vi "solar_excel Worksheet Read (Range).vi"(6 "Truncate Empty Cells? (F)":bool, 8 "error in (no error)":errorcluster, 9 "End (1,1 = 'A1')":cluster{"Row":u32, "Column":u32}, 10 "Start (1,1 = 'A1')":cluster{"Row":u32, "Column":u32}, 11 "Excel Worksheet in":T1) -> (0 "error out":errorcluster, 2 "Cells":string[][](array[string]), 3 "Excel Worksheet out":T1)   [LabVIEW 2018]
doc: "This returns a range of cells from the Worksheet specified by the <b>Start</b> and <b>End</b> cell range."
uses:
  solar_excel_ctl Worksheet.ctl
  solar_excel_ctl TSV.ctl
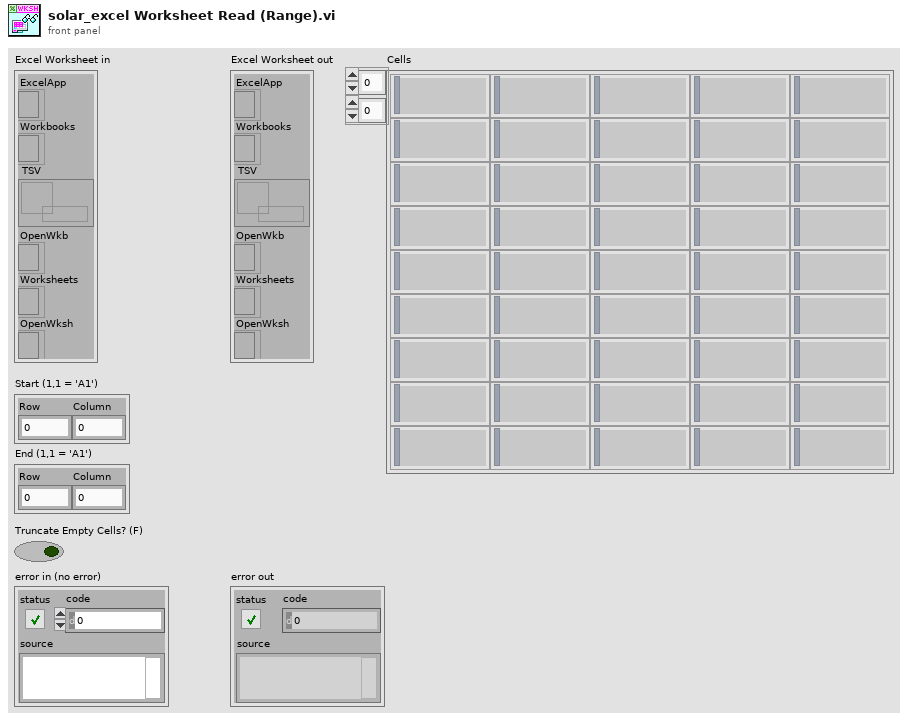
[diagram p1: front panel]
types:
  T1 = typedef "solar_excel_ctl Worksheet.ctl" = cluster{"ExcelApp":refnum<k7>, "Workbooks":refnum<k7>, "TSV":refnum<queue>, "OpenWkb":refnum<k7>, "Worksheets":refnum<k7>, "OpenWksh":refnum<k7>}
  T2 = typedef "solar_excel_ctl TSV.ctl" = cluster{"Path":path, "Dirty":bool, "ActiveSheet":u8, "Worksheets":string[], "Worksheet Cells":cluster{"Cells":string[][]}[]}
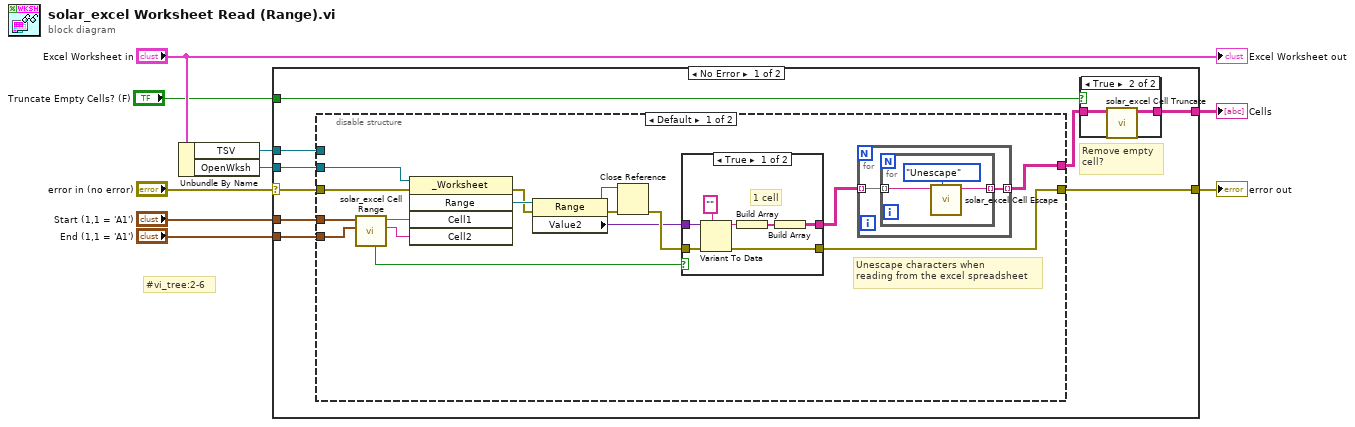
[diagram p0: block diagram]
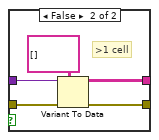
[diagram p2: hidden frame]
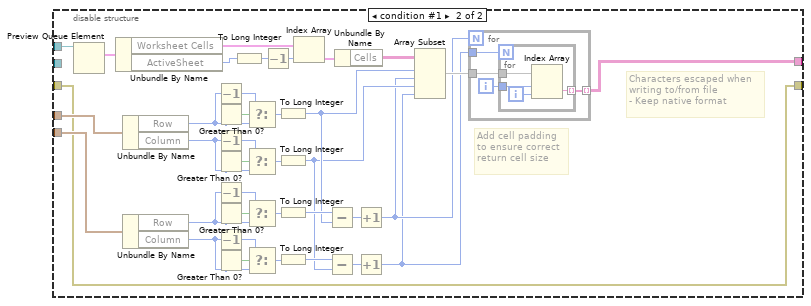
[diagram p3: hidden frame]
diagram:
  # "#vi_tree:2-6"
  n1 = Unbundle By Name("Excel Worksheet in") -> ("TSV"=w1:refnum<queue>, "OpenWksh"=w7:refnum<k7>)
  n2 = case shown="No Error" "error in (no error)" {
    selector: "error in (no error)" -> [w18 w100]
    tunnel: [w16 w100] -> w9
    tunnel: w7 -> [w17 _]
    tunnel: [w13 _] -> w5
    tunnel: "Start (1,1 = 'A1')" -> [w15 _]
    tunnel: "End (1,1 = 'A1')" -> [w14 _]
    tunnel: "Truncate Empty Cells? (F)" -> [w12 _]
    tunnel: w1 -> [w11 _]
    frame No Error {
      # "Remove empty\ncell?"
      n3 = disable-structure shown="Default" {
        disable-tunnel: w18 -> [w33 w56]
        disable-tunnel: w17 -> [w32 _]
        disable-tunnel: [w26 w56] -> w16
        disable-tunnel: w15 -> [w25 w83]
        disable-tunnel: w14 -> [w24 w65]
        disable-tunnel: [w19 w58] -> w10
        disable-tunnel: w11 -> [_ w88]
        frame condition #0 (active) {
          # "Unescape characters when\nreading from the excel spreadsheet"
          n4 = call "solar_excel Cell Range.vi"("End (1,1 = 'A1')"=w24, "Start (1,1 = 'A1')"=w25) -> ("End Cell"=w22:string, "Start Cell"=w23:string, "Same"=w21:bool)  [unwired: 7 in]
          n5 = invoke class="_Worksheet" method="Range"(reference=w32, error in=w33, "Cell1"=w23, "Cell2"=w22) -> (error out=w30:errorcluster, "Range"=w31:refnum<k7>)  [unwired: 1 in, 3 out]
          n6 = property class="Range"(reference=w31, error in=w30) -> (reference out=w28:refnum<k7>, error out=w29:errorcluster, "Value2"=w27:variant)
          n7 = Close Reference(reference=w28, error in (no error)=w29) -> (error out=w34:errorcluster)
          n8 = case shown="True" w21 {
            tunnel: w34 -> [w43 w51]
            tunnel: w27 -> [w44 w50]
            tunnel: [w42 w47] -> w26
            tunnel: [w45 w48] -> w20
            frame True {
              # "1 cell"
              n9 = Variant To Data(error in=w43, type="", Variant=w44) -> (data=w40:string, error out=w42:errorcluster)
              n10 = Build Array(w40) -> (w46:string[])
              n11 = Build Array(w46) -> (w45:string[][])
            }
            frame False {
              # ">1 cell"
              n12 = Variant To Data(error in=w51, type=string[][] [], Variant=w50) -> (data=w48:string[][], error out=w47:errorcluster)
            }
          }
          n13 = for {
            tunnel: w20 -> [w36] mode=indexing
            tunnel: [w35] -> w19 mode=indexing
            n14 = for {
              tunnel: w36 -> [w39] mode=indexing
              tunnel: [w37] -> w35 mode=indexing
              n15 = call "solar_excel Cell Escape.vi"("Action (Escape)"=enum8{"Escape", "Unescape"}."Unescape", "String in"=w39) -> ("String out"=w37:string)  [unwired: 9 in]
            }
          }
        }
        frame condition #1 {
          # "Characters escaped when\nwriting to/from file\n- Keep native format"
          # "Add cell padding\nto ensure correct\nreturn cell size"
          n16 = Preview Queue Element(queue=w88) -> (element=w87:T2)  [unwired: 2 in, 3 out]
          n17 = Unbundle By Name(w87) -> ("Worksheet Cells"=w86:cluster{"Cells":string[][]}[], "ActiveSheet"=w85:u8)
          n18 = Unbundle By Name(w83) -> ("Row"=w79:u32, "Column"=w76:u32)
          n19 = Unbundle By Name(w65) -> ("Row"=w68:u32, "Column"=w71:u32)
          n20 = Decrement(x=w79) -> (x-1=w80:u32)
          n21 = Greater Than 0?(x=w79) -> (x > 0?=w81:bool)
          n22 = Decrement(x=w76) -> (x-1=w78:u32)
          n23 = Greater Than 0?(x=w76) -> (x > 0?=w77:bool)
          n24 = Decrement(x=w68) -> (x-1=w67:u32)
          n25 = Greater Than 0?(x=w68) -> (x > 0?=w66:bool)
          n26 = Decrement(x=w71) -> (x-1=w69:u32)
          n27 = Greater Than 0?(x=w71) -> (x > 0?=w70:bool)
          n28 = To Long Integer(number=w85) -> (32bit integer=w55:i32)
          n29 = Select(t=w80, s=w81, f=w79) -> (s? t:f=w75:u32)
          n30 = Select(t=w78, s=w77, f=w76) -> (s? t:f=w74:u32)
          n31 = Select(t=w67, s=w66, f=w68) -> (s? t:f=w72:u32)
          n32 = Select(t=w69, s=w70, f=w71) -> (s? t:f=w73:u32)
          n33 = Decrement(x=w55) -> (x-1=w54:i32)
          n34 = To Long Integer(number=w75) -> (32bit integer=w63:i32)
          n35 = To Long Integer(number=w74) -> (32bit integer=w61:i32)
          n36 = To Long Integer(number=w72) -> (32bit integer=w64:i32)
          n37 = To Long Integer(number=w73) -> (32bit integer=w62:i32)
          n38 = Index Array(array=w86, index=w54) -> (element=w84:cluster{"Cells":string[][]})
          n39 = Subtract(x=w64, y=w63) -> (x-y=w59:i32)
          n40 = Subtract(x=w62, y=w61) -> (x-y=w57:i32)
          n41 = Unbundle By Name(w84) -> ("Cells"=w82:string[][])
          n42 = Increment(x=w59) -> (x+1=w53:i32)
          n43 = Increment(x=w57) -> (x+1=w52:i32)
          n44 = Array Subset(array=w82, index (row)=w63, length (row)=w53, index (col)=w61, length (col)=w52) -> (w60:string[][])
          n45 = for {
            N: w53 -> [_]
            tunnel: w60 -> [w92]
            tunnel: [w90] -> w58 mode=indexing
            tunnel: w52 -> [w89]
            i -> [w91]
            n46 = for {
              N: w89 -> [_]
              tunnel: w92 -> [w96]
              tunnel: w91 -> [w95]
              tunnel: [w93] -> w90 mode=indexing
              i -> [w94]
              n47 = Index Array(array=w96, index (row)=w95, index (col)=w94) -> (element=w93:string)
            }
          }
        }
      }
      n48 = case shown="True" w12 {
        tunnel: [w97 w99] -> w13
        tunnel: w10 -> [w97 w98]
        frame False {
        }
        frame True {
          n49 = call "solar_excel Cell Truncate.vi"("Cells in"=w98) -> ("Truncated Cells out"=w99:string[][])  [unwired: 10 in]
        }
      }
    }
    frame Error {
    }
  }
  "error out" <- w9
  "Cells" <- w5
  "Excel Worksheet out" <- "Excel Worksheet in"
